vi "net_cycle.vi"() -> ()   [LabVIEW 2020]
doc: "该模板用于创建生产者／消费者模式的应用程序，以事件驱动的方式，生成队列中的项。如需通过响应事件实现代码的异步执行，同时不影响用户界面的响应速度，可考虑用该模式替代“用户界面事件处理器”模式。"
uses:
  6b617843-d38a-4a53-a5bd-3f942f544685.vi
  <vilib>/Instr/_visa.llb/VISA Configure Serial Port (Instr).vi
panel:
  out "开启计时器 3":u32
  out "开启计时器 2":u32
  out "开启计时器":u32
  in  "关时长(ms) 3":u32
  out "数据接收 3":string
  in  "读取的字节 3":i32=500
  in  "远程端口或服务名称 3":u16=29000
  in  "远程主机地址3":string="192.168.76.100"
  in  "关时长(ms) 2":u32
  out "数据接收 2":string
  in  "读取的字节 2":i32=500
  in  "远程端口或服务名称 2":u16=28000
  in  "远程主机地址 2":string="192.168.76.200"
  in  "关时长(ms)":u32
  out "数据接收":string
  out "错误输出":errorcluster
  in  "读取标准码词":bool
  out "读取标准码词":string
  in  "发送数据(十六进制)":string="\u0001T\u0004"
  in  "读取的字节":i32=500
  in  "远程端口或服务名称":u16=30000
  in  "远程主机地址":string="192.168.76.172"
  in  "压缩机":bool
  in  "臭氧\n臭氧":bool
  in  "开时长(ms)":u32
  in  "开时长(ms) 2":u32
  in  "开时长(ms)  3":u32
  in  "开始测试":bool
  in  "风机":bool
  out "error out":errorcluster caption="继电器板错误输入输出"
  in  "继电器调试":bool
  in  "打开开关":bool
  in  "串口资源":refnum<visa-resource-name>
  in  "stop":bool caption="停止"
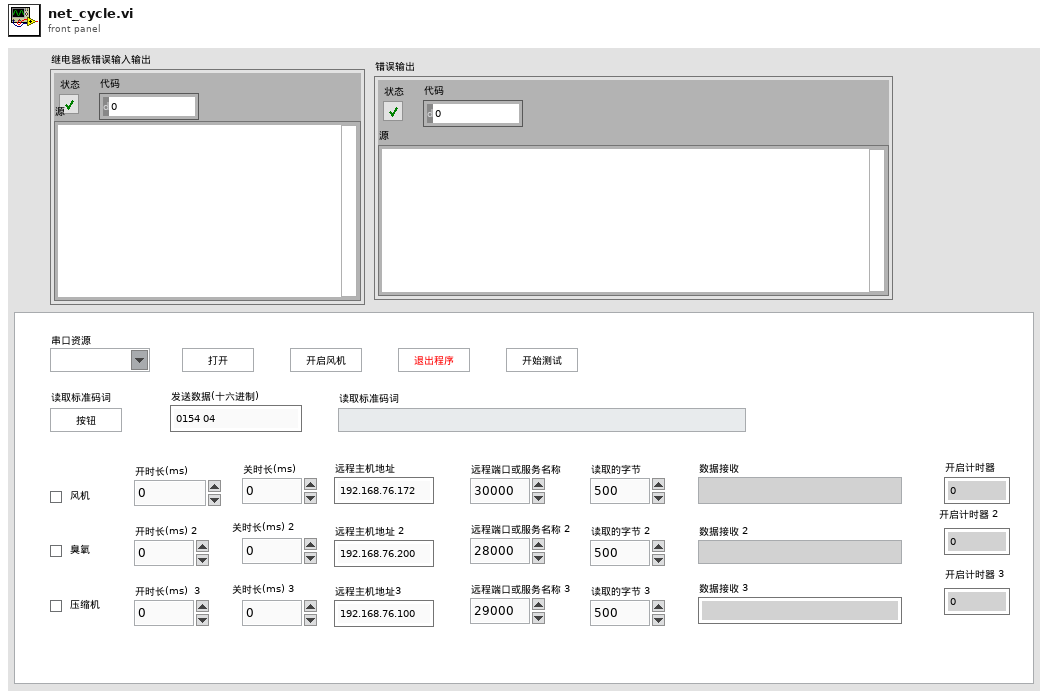
[diagram p1: front panel]
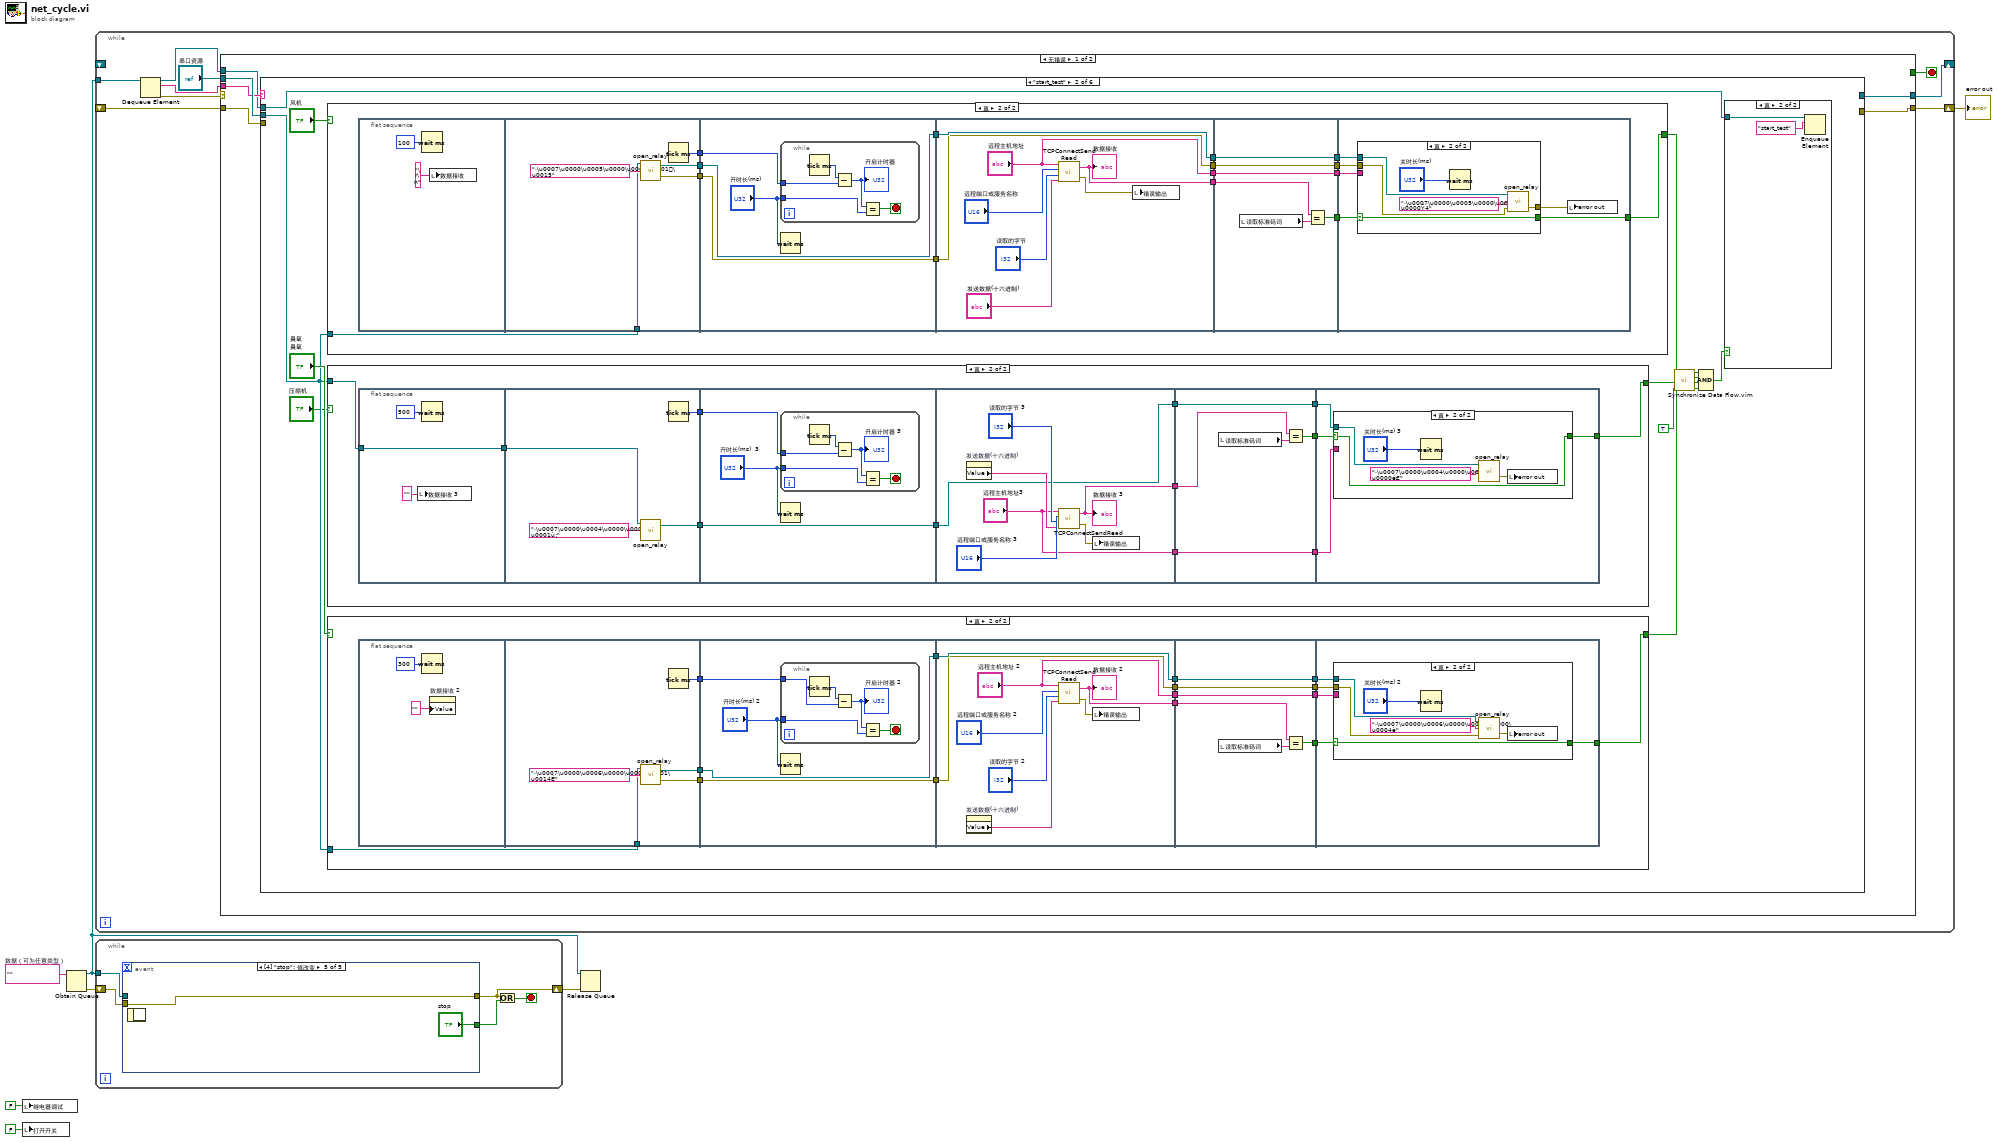
[diagram p0: block diagram]
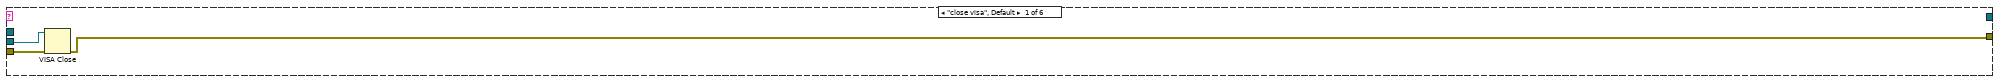
[diagram p2: hidden frame]
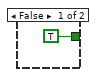
[diagram p4: hidden frame]
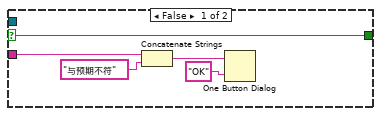
[diagram p5: hidden frame]
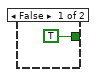
[diagram p6: hidden frame]
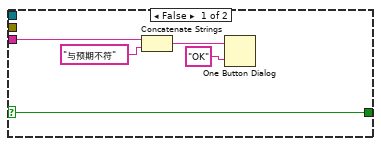
[diagram p7: hidden frame]
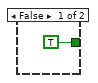
[diagram p8: hidden frame]
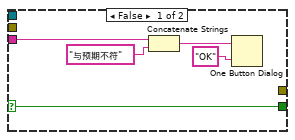
[diagram p9: hidden frame]
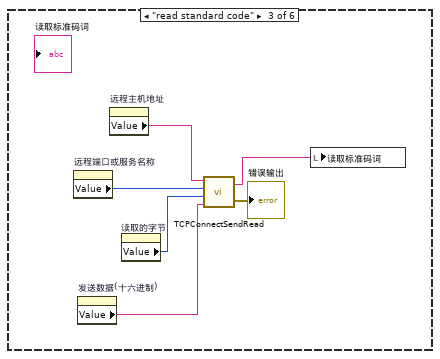
[diagram p10: hidden frame]
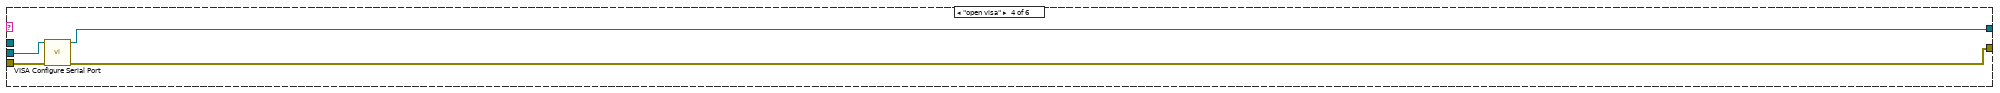
[diagram p11: hidden frame]
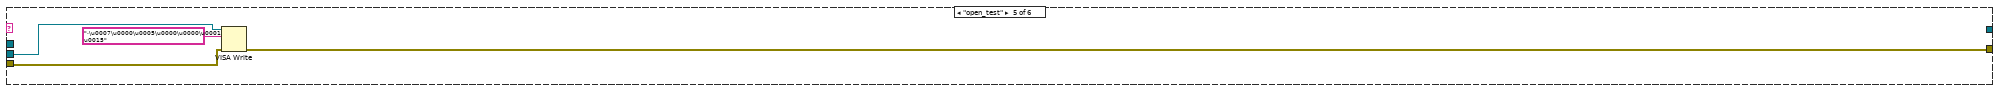
[diagram p12: hidden frame]
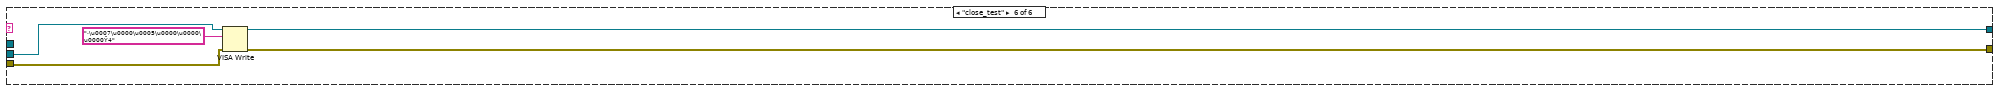
[diagram p13: hidden frame]
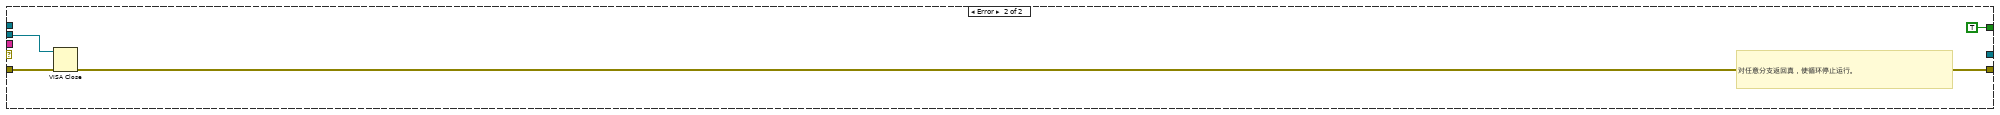
[diagram p14: hidden frame]
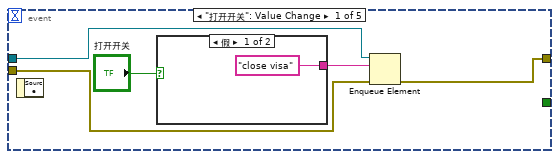
[diagram p15: hidden frame]
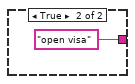
[diagram p16: hidden frame]
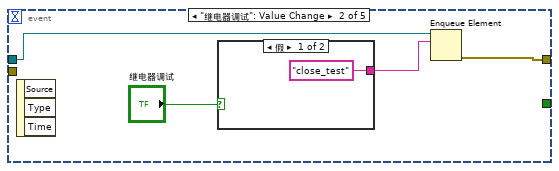
[diagram p17: hidden frame]
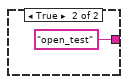
[diagram p18: hidden frame]
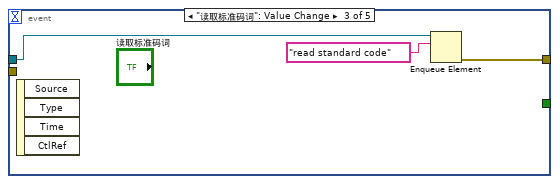
[diagram p19: hidden frame]
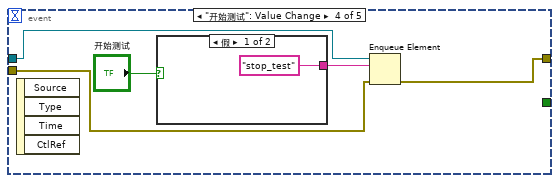
[diagram p20: hidden frame]
diagram:
  w5 = ""  # 数据（可为任意类型）
  n1 = local write "继电器调试"(FALSE ("继电器调试")) -> ()
  n2 = local write "打开开关"(FALSE ("打开开关")) -> ()
  n3 = Obtain Queue(element data type=w5) -> (queue out=w4:refnum<queue>, error out=w7:errorcluster)  [unwired: 4 in, 1 out]
  n4 = while {
    tunnel: w4 -> [w16]
    shift-right: [w12] -> _
    shift-left: _ -> [_]
    shift-right: [w11] -> w3
    shift-left: _ -> [w10]
    stop <- w15 stop-if-true
    n5 = Dequeue Element(queue=w16) -> (queue out=w8:refnum<queue>, element=w13:string, error out=w14:errorcluster)  [unwired: 2 in, 1 out]
    n6 = case shown="无错误" w14 {
      tunnel: [_ TRUE] -> w15
      tunnel: w13 -> [w18 _]
      tunnel: [w22 _] -> w12
      tunnel: "串口资源" -> [w21 w242]
      tunnel: [w19 w240] -> w11
      tunnel: w10 -> [w20 w241]
      tunnel: w8 -> [w17 _]
      frame No Error {
        n7 = case shown="\"start_test\"" w18 {
          tunnel: [_ _ _ w230 _ w236] -> w22
          tunnel: w21 -> [w25 w37 _ w227 w234 w237]
          tunnel: w20 -> [w24 _ _ w228 w231 w235]
          tunnel: [w23 _ _ w229 w232 w239] -> w19
          tunnel: w17 -> [_ w30 _ _ _ _]
          frame "close visa", Default {
            n8 = VISA Close(VISA resource name=w25, error in (no error)=w24) -> (error out=w23:errorcluster)
          }
          frame "start_test" {
            n9 = case shown="真" "风机" {
              tunnel: w37 -> [_ w173]
              tunnel: [TRUE w168] -> w35
              frame False {
              }
              frame True {
                n10 = flat-sequence {
                  tunnel: w173 -> [w179]
                  tunnel: [w178] -> w167
                  tunnel: [w177] -> w163
                  tunnel: [w176] -> w159
                  tunnel: w167 -> [w184]
                  tunnel: [w184] -> w166
                  tunnel: w163 -> [w183]
                  tunnel: [w183] -> w162
                  tunnel: w159 -> [w182]
                  tunnel: [w194] -> w172
                  tunnel: w166 -> [w193]
                  tunnel: [w193] -> w171
                  tunnel: ["远程主机地址"] -> w164
                  tunnel: w162 -> [w191]
                  tunnel: [w191] -> w161
                  tunnel: w172 -> [w203]
                  tunnel: w171 -> [w201]
                  tunnel: [w201] -> w170
                  tunnel: [w200] -> w169
                  tunnel: [w199] -> w165
                  tunnel: w164 -> [w199]
                  tunnel: w161 -> [w198]
                  tunnel: [w198] -> w160
                  tunnel: w170 -> [w209]
                  tunnel: w169 -> [w208]
                  tunnel: [w207] -> w168
                  tunnel: w165 -> [w206]
                  tunnel: w160 -> [w205]
                  frame #0 {
                    n11 = Wait (ms)(milliseconds to wait=u32 100 ("等待时间（毫秒）")) -> ()  [unwired: 1 out]
                    n12 = local write "数据接收"("\r\n" ("数据接收")) -> ()
                  }
                  frame #1 {
                    n13 = call "open_relay.vi"("写入缓冲区"="·\u0007\u0000\u0005\u0000\u0000\u0001\u0015", "VISA资源名称"=w179) -> ("错误输出"=w177:errorcluster, "VISA资源名称输出"=w178:refnum<visa-resource-name>)  [unwired: 1 in]
                    n14 = Tick Count (ms)() -> (millisecond timer value=w176:u32)
                  }
                  frame #2 {
                    n15 = while {
                      tunnel: w182 -> [w188]
                      tunnel: "开时长(ms)" -> [w185]
                      stop <- w187 stop-if-true
                      n16 = Tick Count (ms)() -> (millisecond timer value=w189:u32)
                      n17 = Subtract(x=w189, y=w188) -> (x-y=w186:u32)
                      "开启计时器" <- w186
                      n18 = Equal?(x=w186, y=w185) -> (x = y?=w187:bool)
                    }
                    n19 = Wait (ms)(milliseconds to wait="开时长(ms)") -> ()  [unwired: 1 out]
                  }
                  frame #3 {
                    n20 = call "TCPConnectSendRead.vi"("数据输入"="发送数据(十六进制)", "读取的字节"="读取的字节", "远程端口或服务名称"="远程端口或服务名称", "地址"="远程主机地址") -> ("错误输出"=w190:errorcluster, "数据输出"=w194:string)
                    "数据接收" <- w194
                    n21 = local write "错误输出"(w190) -> ()
                  }
                  frame #4 {
                    n22 = local read "读取标准码词"() -> (w202:string)
                    n23 = Equal?(x=w203, y=w202) -> (x = y?=w200:bool)
                  }
                  frame #5 {
                    n24 = case shown="真" w208 {
                      selector: w208 -> [w214 w217]
                      tunnel: w209 -> [_ w219]
                      tunnel: [w214 w217] -> w207
                      tunnel: w206 -> [w212 _]
                      tunnel: w205 -> [_ w216]
                      tunnel: [_ w215] -> w204
                      frame False {
                        n25 = Concatenate Strings(w212, "与预期不符" ("字符串")) -> (w210:string)
                        n26 = One Button Dialog(message=w210, button name ("OK")="OK" ("按钮名称（“确定”）")) -> ()  [unwired: 1 out]
                      }
                      frame True {
                        n27 = Wait (ms)(milliseconds to wait="关时长(ms)") -> ()  [unwired: 1 out]
                        n28 = call "open_relay.vi"("错误输入（无错误）"=w216, "写入缓冲区"="·\u0007\u0000\u0005\u0000\u0000\u0000Ÿ4", "VISA资源名称"=w219) -> ("错误输出"=w215:errorcluster)  [unwired: 1 out]
                      }
                    }
                    n29 = local write "error out"(w204) -> ()
                  }
                }
              }
            }
            n30 = case shown="真" "压缩机" {
              tunnel: w37 -> [_ w53]
              tunnel: [TRUE w48] -> w29
              frame False {
              }
              frame True {
                n31 = flat-sequence {
                  tunnel: w53 -> [w57]
                  tunnel: [w57] -> w54
                  tunnel: w54 -> [w61]
                  tunnel: [w59] -> w44
                  tunnel: [w58] -> w43
                  tunnel: [w64] -> w45
                  tunnel: w44 -> [w64]
                  tunnel: w43 -> [w63]
                  tunnel: [w72] -> w52
                  tunnel: ["远程主机地址3"] -> w49
                  tunnel: [w70] -> w46
                  tunnel: w45 -> [w70]
                  tunnel: w52 -> [w81]
                  tunnel: [w79] -> w51
                  tunnel: [w78] -> w50
                  tunnel: w49 -> [w78]
                  tunnel: [w77] -> w47
                  tunnel: w46 -> [w77]
                  tunnel: w51 -> [w85]
                  tunnel: w50 -> [w84]
                  tunnel: [w83] -> w48
                  tunnel: w47 -> [w82]
                  frame #0 {
                    n32 = local write "数据接收 3"("" ("数据接收 3")) -> ()
                    n33 = Wait (ms)(milliseconds to wait=u32 500 ("等待时间（毫秒）")) -> ()  [unwired: 1 out]
                  }
                  frame #1 {
                    n34 = call "open_relay.vi"("写入缓冲区"="·\u0007\u0000\u0004\u0000\u0000\u0001ù¡", "VISA资源名称"=w61) -> ("VISA资源名称输出"=w59:refnum<visa-resource-name>)  [unwired: 1 in, 1 out]
                    n35 = Tick Count (ms)() -> (millisecond timer value=w58:u32)
                  }
                  frame #2 {
                    n36 = while {
                      tunnel: w63 -> [w67]
                      tunnel: "开时长(ms)  3" -> [w66]
                      stop <- w68 stop-if-true
                      n37 = Tick Count (ms)() -> (millisecond timer value=w69:u32)
                      n38 = Subtract(x=w69, y=w67) -> (x-y=w65:u32)
                      "开启计时器 3" <- w65
                      n39 = Equal?(x=w65, y=w66) -> (x = y?=w68:bool)
                    }
                    n40 = Wait (ms)(milliseconds to wait="开时长(ms)  3") -> ()  [unwired: 1 out]
                  }
                  frame #3 {
                    n41 = property on="发送数据(十六进制)" class="Str"() -> ("Value"=w74:string)  [unwired: 2 in, 2 out]
                    n42 = call "TCPConnectSendRead.vi"("数据输入"=w74, "读取的字节"="读取的字节 3", "远程端口或服务名称"="远程端口或服务名称 3", "地址"="远程主机地址3") -> ("错误输出"=w73:errorcluster, "数据输出"=w72:string)
                    "数据接收 3" <- w72
                    n43 = local write "错误输出"(w73) -> ()
                  }
                  frame #4 {
                    n44 = local read "读取标准码词"() -> (w80:string)
                    n45 = Equal?(x=w81, y=w80) -> (x = y?=w79:bool)
                  }
                  frame #5 {
                    n46 = case shown="真" w85 {
                      selector: w85 -> [w86 w92]
                      tunnel: w84 -> [w87 _]
                      tunnel: [w86 w92] -> w83
                      tunnel: w82 -> [_ w91]
                      frame False {
                        n47 = Concatenate Strings(w87, "与预期不符" ("字符串")) -> (w88:string)
                        n48 = One Button Dialog(message=w88, button name ("OK")="OK" ("按钮名称（“确定”）")) -> ()  [unwired: 1 out]
                      }
                      frame True {
                        n49 = Wait (ms)(milliseconds to wait="关时长(ms) 3") -> ()  [unwired: 1 out]
                        n50 = call "open_relay.vi"("写入缓冲区"="·\u0007\u0000\u0004\u0000\u0000\u0000é€", "VISA资源名称"=w91) -> ("错误输出"=w94:errorcluster)  [unwired: 1 in, 1 out]
                        n51 = local write "error out"(w94) -> ()
                      }
                    }
                  }
                }
              }
            }
            n52 = case shown="真" "臭氧\n臭氧" {
              tunnel: w37 -> [_ w111]
              tunnel: [TRUE w98] -> w34
              frame False {
              }
              frame True {
                n53 = flat-sequence {
                  tunnel: w111 -> [w117]
                  tunnel: [w116] -> w110
                  tunnel: [w115] -> w102
                  tunnel: [w114] -> w97
                  tunnel: w110 -> [w122]
                  tunnel: [w122] -> w109
                  tunnel: [w121] -> w103
                  tunnel: w102 -> [w121]
                  tunnel: w97 -> [w120]
                  tunnel: w109 -> [w135]
                  tunnel: [w135] -> w108
                  tunnel: [w132] -> w107
                  tunnel: [w131] -> w104
                  tunnel: w103 -> [w131]
                  tunnel: ["远程主机地址 2"] -> w100
                  tunnel: w108 -> [w139]
                  tunnel: w107 -> [w141]
                  tunnel: [w139] -> w106
                  tunnel: [w138] -> w105
                  tunnel: w104 -> [w138]
                  tunnel: [w137] -> w101
                  tunnel: w100 -> [w137]
                  tunnel: [w136] -> w99
                  tunnel: w106 -> [w146]
                  tunnel: w105 -> [w145]
                  tunnel: w101 -> [w144]
                  tunnel: w99 -> [w143]
                  tunnel: [w142] -> w98
                  frame #0 {
                    n54 = Wait (ms)(milliseconds to wait=u32 300 ("等待时间（毫秒）")) -> ()  [unwired: 1 out]
                    n55 = property on="数据接收 2" class="Str"("Value"="" ("数据接收 2")) -> ()  [unwired: 2 in, 2 out]
                  }
                  frame #1 {
                    n56 = call "open_relay.vi"("写入缓冲区"="·\u0007\u0000\u0006\u0000\u0000\u0001\u0014É", "VISA资源名称"=w117) -> ("错误输出"=w115:errorcluster, "VISA资源名称输出"=w116:refnum<visa-resource-name>)  [unwired: 1 in]
                    n57 = Tick Count (ms)() -> (millisecond timer value=w114:u32)
                  }
                  frame #2 {
                    n58 = while {
                      tunnel: w120 -> [w125]
                      tunnel: "开时长(ms) 2" -> [w124]
                      stop <- w126 stop-if-true
                      n59 = Tick Count (ms)() -> (millisecond timer value=w127:u32)
                      n60 = Subtract(x=w127, y=w125) -> (x-y=w123:u32)
                      "开启计时器 2" <- w123
                      n61 = Equal?(x=w123, y=w124) -> (x = y?=w126:bool)
                    }
                    n62 = Wait (ms)(milliseconds to wait="开时长(ms) 2") -> ()  [unwired: 1 out]
                  }
                  frame #3 {
                    n63 = property on="发送数据(十六进制)" class="Str"() -> ("Value"=w130:string)  [unwired: 2 in, 2 out]
                    n64 = call "TCPConnectSendRead.vi"("数据输入"=w130, "读取的字节"="读取的字节 2", "远程端口或服务名称"="远程端口或服务名称 2", "地址"="远程主机地址 2") -> ("错误输出"=w128:errorcluster, "数据输出"=w132:string)
                    "数据接收 2" <- w132
                    n65 = local write "错误输出"(w128) -> ()
                  }
                  frame #4 {
                    n66 = local read "读取标准码词"() -> (w140:string)
                    n67 = Equal?(x=w141, y=w140) -> (x = y?=w136:bool)
                  }
                  frame #5 {
                    n68 = case shown="真" w143 {
                      selector: w143 -> [w147 w152]
                      tunnel: w146 -> [_ w156]
                      tunnel: w145 -> [_ w155]
                      tunnel: w144 -> [w148 _]
                      tunnel: [w147 w152] -> w142
                      frame False {
                        n69 = Concatenate Strings(w148, "与预期不符" ("字符串")) -> (w151:string)
                        n70 = One Button Dialog(message=w151, button name ("OK")="OK" ("按钮名称（“确定”）")) -> ()  [unwired: 1 out]
                      }
                      frame True {
                        n71 = Wait (ms)(milliseconds to wait="关时长(ms) 2") -> ()  [unwired: 1 out]
                        n72 = call "open_relay.vi"("错误输入（无错误）"=w155, "写入缓冲区"="·\u0007\u0000\u0006\u0000\u0000\u0000\u0004è", "VISA资源名称"=w156) -> ("错误输出"=w154:errorcluster)  [unwired: 1 out]
                        n73 = local write "error out"(w154) -> ()
                      }
                    }
                  }
                }
              }
            }
            n74 = call "Synchronize Data Flow.vim"("input 4"=TRUE, "input 3"=w29, "input 2"=w34, "input 1"=w35) -> ("output 4"=w26:bool, "output 3"=w28:bool, "output 2"=w32:bool, "output 1"=w33:bool)
            n75 = Compound Arithmetic op=AND ("复合运算")(w33, w32, w28, w26) -> (w31:bool)
            n76 = case shown="真" w31 {
              tunnel: w30 -> [_ w40]
              frame False {
              }
              frame True {
                n77 = Enqueue Element(queue=w40, element="start_test" ("元素")) -> ()  [unwired: 2 in, 3 out]
              }
            }
          }
          frame "read standard code" {
            n78 = property on="远程端口或服务名称" class="DigNum (严格)"() -> ("Value"=w225:u16)  [unwired: 2 in, 2 out]
            n79 = property on="发送数据(十六进制)" class="Str"() -> ("Value"=w223:string)  [unwired: 2 in, 2 out]
            n80 = property on="远程主机地址" class="Str"() -> ("Value"=w224:string)  [unwired: 2 in, 2 out]
            n81 = property on="读取的字节" class="DigNum (严格)"() -> ("Value"=w226:i32)  [unwired: 2 in, 2 out]
            n82 = call "TCPConnectSendRead.vi"("数据输入"=w223, "读取的字节"=w226, "远程端口或服务名称"=w225, "地址"=w224) -> ("错误输出"=→"错误输出":errorcluster, "数据输出"=w222:string)
            n83 = local write "读取标准码词"(w222) -> ()
          }
          frame "open visa" {
            n84 = call-poly "VISA Configure Serial Port"("VISA resource name"=w227, "error in (no error)"=w228) -> ("VISA resource name out"=w230:refnum<visa-resource-name>, "error out"=w229:errorcluster)  [unwired: 12 in]
          }
          frame "open_test" {
            n85 = VISA Write(VISA resource name=w234, write buffer="·\u0007\u0000\u0005\u0000\u0000\u0001\u0015" ("写入缓冲区"), error in (no error)=w231) -> (error out=w232:errorcluster)  [unwired: 2 out]
          }
          frame "close_test" {
            n86 = VISA Write(VISA resource name=w237, write buffer="·\u0007\u0000\u0005\u0000\u0000\u0000Ÿ4" ("写入缓冲区"), error in (no error)=w235) -> (VISA resource name out=w236:refnum<visa-resource-name>, error out=w239:errorcluster)  [unwired: 1 out]
          }
        }
      }
      frame Error {
        # "对任意分支返回真，使循环停止运行。"
        n87 = VISA Close(VISA resource name=w242, error in (no error)=w241) -> (error out=w240:errorcluster)
      }
    }
  }
  "error out" <- w3
  n88 = while {
    shift-right: [w244] -> w6
    shift-left: w7 -> [w247]
    tunnel: w4 -> [w248]
    stop <- w245 stop-if-true
    n89 = event shown="[4] \"stop\": 值改变" {
      selector: _ -> [_ _ _ _ _]
      dyn-events: _ -> [_ _ _ _ _]
      timeout: _ -> [_ _ _ _ _]
      tunnel: w248 -> [w253 w258 w264 w267 _]
      tunnel: w247 -> [w252 _ _ w268 w272]
      tunnel: [w251 w259 w263 w269 w272] -> w244
      tunnel: [_ _ _ _ "stop"] -> w246
      event "打开开关": Value Change {
        n90 = event-data() -> ()  [unwired: 1 in, 1 out]
        n91 = case shown="假" "打开开关" {
          tunnel: ["close visa" ("element") "open visa" ("element")] -> w249
          frame False {
          }
          frame True {
          }
        }
        n92 = Enqueue Element(queue=w253, element=w249, error in (no error)=w252) -> (error out=w251:errorcluster)  [unwired: 1 in, 2 out]
      }
      event "继电器调试": Value Change {
        n93 = event-data() -> ()  [unwired: 1 in, 3 out]
        n94 = case shown="假" "继电器调试" {
          tunnel: ["close_test" ("元素") "open_test" ("元素")] -> w256
          frame False {
          }
          frame True {
          }
        }
        n95 = Enqueue Element(queue=w258, element=w256) -> (error out=w259:errorcluster)  [unwired: 2 in, 2 out]
      }
      event "读取标准码词": Value Change {
        n96 = event-data() -> ()  [unwired: 1 in, 4 out]
        n97 = Enqueue Element(queue=w264, element="read standard code" ("元素")) -> (error out=w263:errorcluster)  [unwired: 2 in, 2 out]
      }
      event "开始测试": Value Change {
        n98 = event-data() -> ()  [unwired: 1 in, 4 out]
        n99 = case shown="假" "开始测试" {
          tunnel: ["stop_test" ("元素") "start_test" ("元素")] -> w265
          frame False {
          }
          frame True {
          }
        }
        n100 = Enqueue Element(queue=w267, element=w265, error in (no error)=w268) -> (error out=w269:errorcluster)  [unwired: 1 in, 2 out]
      }
      event "stop": Value Change {
        n101 = event-data() -> ()  [unwired: 1 in, 1 out]
      }
    }
    n102 = Or(x=w244, y=w246) -> (x .or. y?=w245:bool)
  }
  n103 = Release Queue(queue=w4, error in (no error)=w6) -> ()  [unwired: 1 in, 3 out]
